vi "TestBuildPISLoop.vi"(8 "error in (no error)":errorcluster) -> (0 "error out":errorcluster)   [LabVIEW 2019]
uses:
  <vilib>/addons/_JKI Toolkits/Caraya/classes/Test/Test.lvclass
  <vilib>/addons/_JKI Toolkits/Caraya/classes/Assert/Assert.lvclass
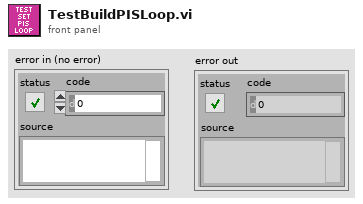
[diagram p1: front panel]
types:
  T1 = cluster{"setpoint":dbl, "pgain":dbl, "igain":dbl, "sgain":dbl}
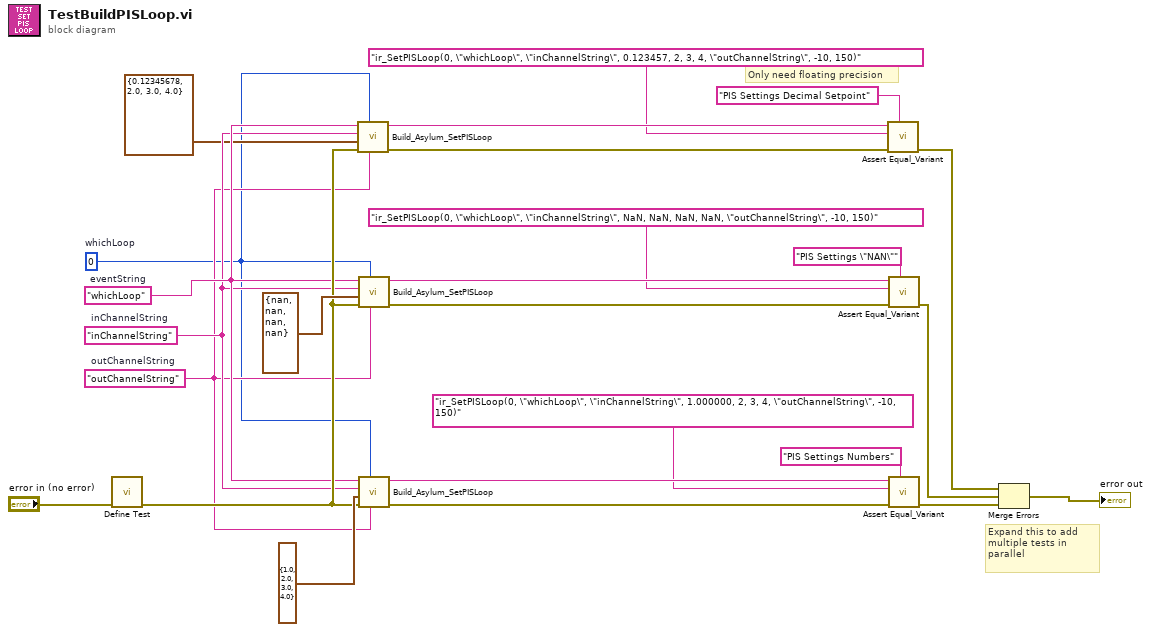
[diagram p0: block diagram]
diagram:
  w6 = "outChannelString"  # outChannelString
  w7 = "inChannelString"  # inChannelString
  w8 = "whichLoop"  # eventString
  w4 = 0  # whichLoop
  # "Only need floating precision"
  # "Expand this to add multiple tests in parallel"
  n1 = call <vilib>:"Define Test.vi"("error in (no error)"="error in (no error)") -> ("error out"=w9:errorcluster)  [unwired: 10 in]
  n2 = call "Build_Asylum_SetPISLoop.vi"("outChannelString"=w6, "whichLoop"=w4, "error in (no error)"=w9, "PIS Controls"=T1 {"setpoint"=0.12345678, "pgain"=2.0, "igain"=3.0, "sgain"=4.0}, "inChannelString"=w7, "eventString"=w8) -> ("error out"=w10:errorcluster, "Command"=w3:string)  [unwired: 4 in]
  n3 = call "Build_Asylum_SetPISLoop.vi"("outChannelString"=w6, "whichLoop"=w4, "error in (no error)"=w9, "PIS Controls"=T1 {"setpoint"=nan, "pgain"=nan, "igain"=nan, "sgain"=nan}, "inChannelString"=w7, "eventString"=w8) -> ("error out"=w17:errorcluster, "Command"=w18:string)  [unwired: 4 in]
  n4 = call "Build_Asylum_SetPISLoop.vi"("outChannelString"=w6, "whichLoop"=w4, "error in (no error)"=w9, "PIS Controls"=T1 {"setpoint"=1.0, "pgain"=2.0, "igain"=3.0, "sgain"=4.0}, "inChannelString"=w7, "eventString"=w8) -> ("error out"=w21:errorcluster, "Command"=w20:string)  [unwired: 4 in]
  n5 = call <vilib>:"Assert Equal_Variant.vi"("Label"="PIS Settings Decimal Setpoint", "error in (no error)"=w10, "Y"="ir_SetPISLoop(0, \"whichLoop\", \"inChannelString\", 0.123457, 2, 3, 4, \"outChannelString\", -10, 150)", "X"=w3) -> ("error out"=w11:errorcluster)  [unwired: 7 in]
  n6 = call <vilib>:"Assert Equal_Variant.vi"("Label"="PIS Settings \"NAN\"", "error in (no error)"=w17, "Y"="ir_SetPISLoop(0, \"whichLoop\", \"inChannelString\", NaN, NaN, NaN, NaN, \"outChannelString\", -10, 150)", "X"=w18) -> ("error out"=w15:errorcluster)  [unwired: 7 in]
  n7 = call <vilib>:"Assert Equal_Variant.vi"("Label"="PIS Settings Numbers", "error in (no error)"=w21, "Y"="ir_SetPISLoop(0, \"whichLoop\", \"inChannelString\", 1.000000, 2, 3, 4, \"outChannelString\", -10, 150)", "X"=w20) -> ("error out"=w23:errorcluster)  [unwired: 7 in]
  n8 = Merge Errors(w11, w15, w23) -> (→"error out":errorcluster)
